vi "Val to angle right.vi"(11 "Sensor val":dbl) -> (3 "Right bending angle":dbl format="%_6f")   [LabVIEW 2019]
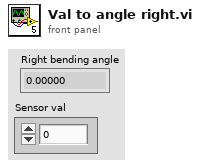
[diagram p1: front panel]
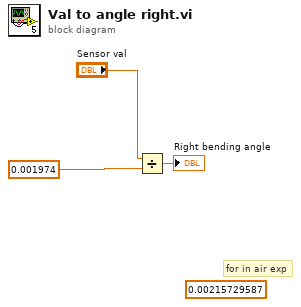
[diagram p0: block diagram]
diagram:
  (unwired) 0.00215729587
  # "for in air exp"
  n1 = Divide(x="Sensor val", y=0.001974) -> (x/y=→"Right bending angle":dbl)
